vi "Open System Definition.vi"(8 "error in (no error)":errorcluster, 11 "System Definition File":path) -> (0 "error out":errorcluster, 1 "Target Refnum":refnum<k24>, 2 "Root Refnum":refnum<k24>, 3 "System Definition Refnum":refnum<k24>)   [LabVIEW 2018, in "Instrument Addon Scripting API.lvlib"]
uses:
  Instrument Addon Scripting API.lvlib
  NationalInstruments.VeriStand.SystemDefinitionAPI
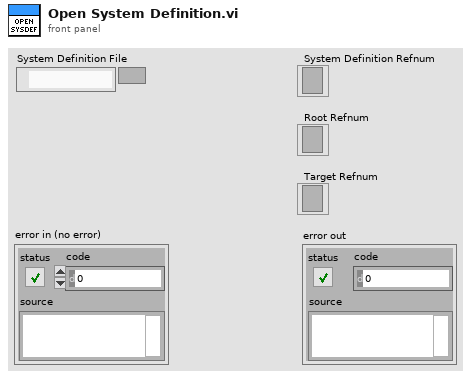
[diagram p1: front panel]
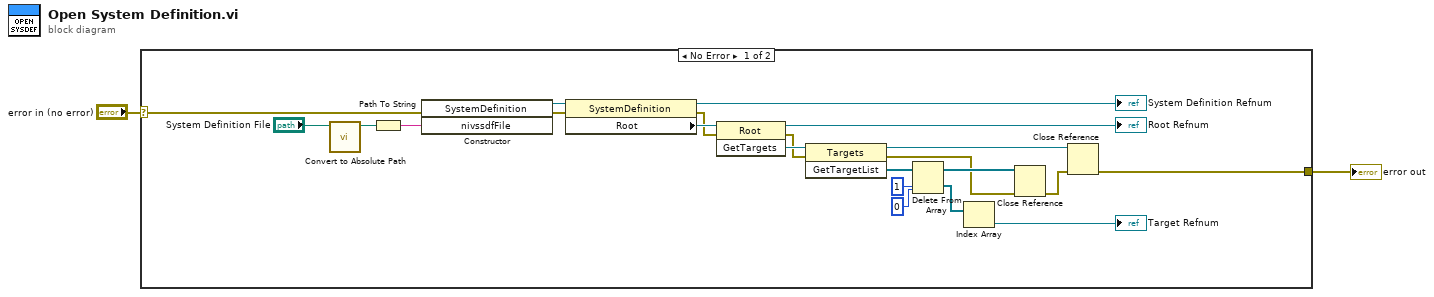
[diagram p0: block diagram]
diagram:
  n1 = case shown="No Error" "error in (no error)" {
    selector: "error in (no error)" -> [w5 w25]
    tunnel: [w4 w25] -> w1
    frame No Error {
      n2 = call "Convert to Absolute Path.vi"("System Definition File"="System Definition File") -> ("Absolute Path"=w6:path)  [unwired: 10 in]
      n3 = Path To String(path=w6) -> (string=w7:string)
      n4 = constructor class="SystemDefinition"(error in=w5, "nivssdfFile"=w7) -> (reference out=w9:refnum<k24>, error out=w8:errorcluster)  [unwired: 2 in, 2 out]
      n5 = property class="SystemDefinition"(reference=w9, error in=w8) -> (reference out=→"System Definition Refnum":refnum<k24>, error out=w10:errorcluster, "Root"=w11:refnum<k24>)
      n6 = invoke class="Root" method="GetTargets"(reference=w11, error in=w10) -> (reference out=→"Root Refnum":refnum<k24>, error out=w12:errorcluster, "GetTargets"=w13:refnum<k24>)  [unwired: 1 in]
      n7 = invoke class="Targets" method="GetTargetList"(reference=w13, error in=w12) -> (reference out=w20:refnum<k24>, error out=w17:errorcluster, "GetTargetList"=w14:refnum<k24>[])  [unwired: 1 in]
      n8 = Delete From Array(array=w14, length=1, index=0) -> (deleted portion=w21:refnum<k24>[], array with subset deleted=w18:refnum<k24>[])
      n9 = Index Array(array=w21) -> (element=→"Target Refnum":refnum<k24>)  [unwired: 1 in]
      n10 = Close Reference(reference=w18, error in (no error)=w17) -> (error out=w19:errorcluster)
      n11 = Close Reference(reference=w20, error in (no error)=w19) -> (error out=w4:errorcluster)
    }
    frame Error {
    }
  }
  "error out" <- w1
